vi "gugudan server.vi"() -> ()   [LabVIEW 2014]
uses:
  <vilib>/FTP/NI_FTP.lvlib
panel:
  in  "data 2":string="연결된 IP"
  in  "숫자형":dbl min=0.0 max=24.0 step=0.5
  in  "재시작":bool
  in  "2시간":bool
  in  "강제종료":bool
  in  "1시간":bool
  in  "종료취소":bool
  in  "종료":bool
  out "data":string="연결된 IP"
  in  "사용설명서":bool
  out "로그인":bool
  in  "ID":string="ID"
  in  "PW":string="PW"
  in  "E-Mail":string="E-Mail  address"
  out "참 거짓":string="상태창입니다."
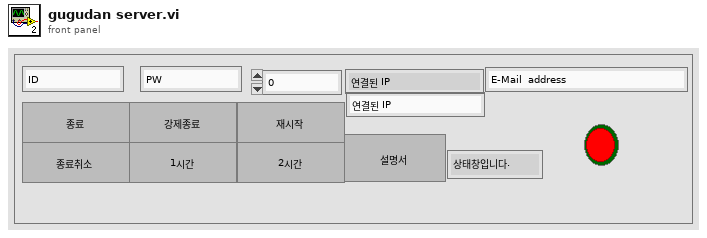
[diagram p1: front panel]
types:
  T1 = typedef "NI_FTP.lvlib/FTP Session.ctl" = refnum<k5>
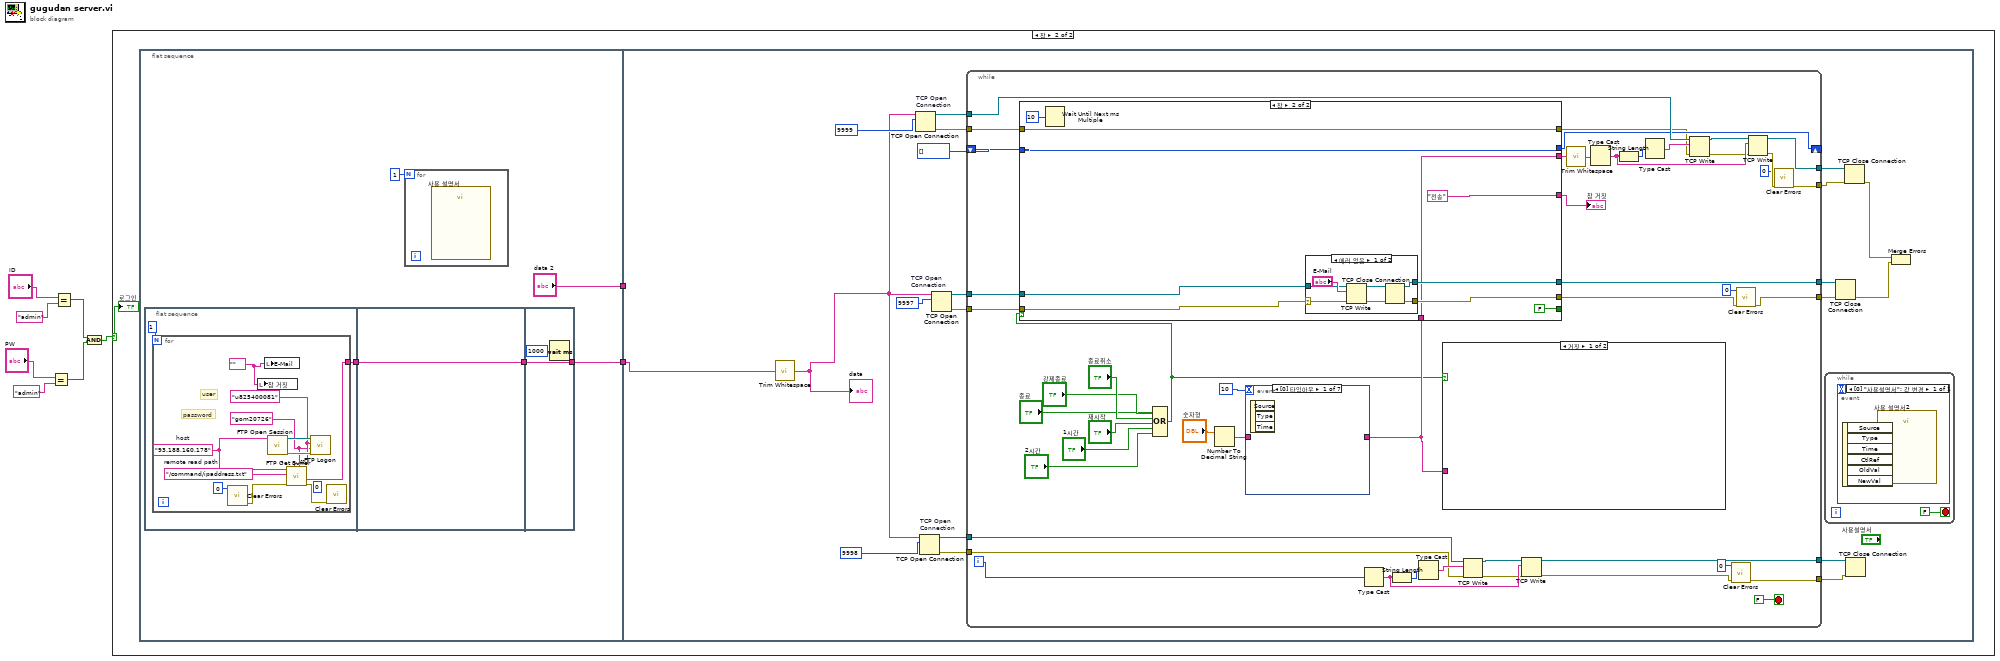
[diagram p0: block diagram]
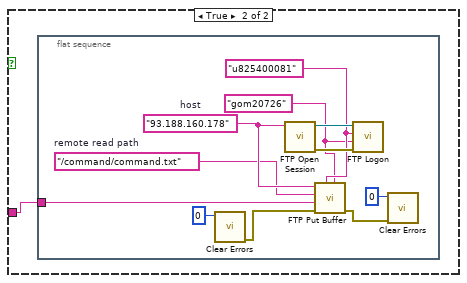
[diagram p3: hidden frame]
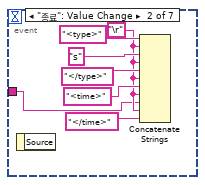
[diagram p4: hidden frame]
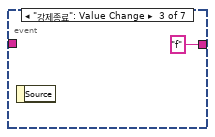
[diagram p5: hidden frame]
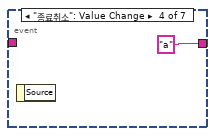
[diagram p6: hidden frame]
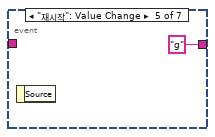
[diagram p7: hidden frame]
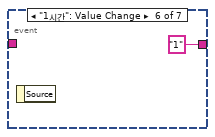
[diagram p8: hidden frame]
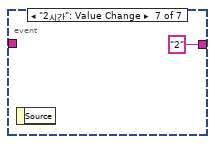
[diagram p9: hidden frame]
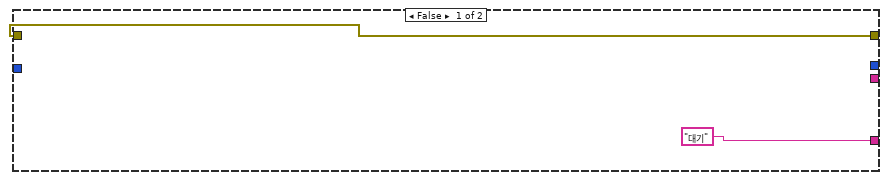
[diagram p10: hidden frame]
diagram:
  n1 = Equal?(x="PW", y="admin") -> (x = y?=w2:bool)
  n2 = Equal?(x="ID", y="admin") -> (x = y?=w3:bool)
  n3 = And(x=w3, y=w2) -> (x .and. y?=w1:bool)
  n4 = case shown="참" w1 {
    selector: w1 -> [_ w9]
    frame False {
    }
    frame True {
      n5 = flat-sequence {
        tunnel: [w14] -> w10
        tunnel: ["data 2"] -> w8
        tunnel: w10 -> [w32]
        tunnel: w8 -> [_]
        frame #0 {
          n6 = flat-sequence {
            tunnel: [w17] -> w13
            tunnel: w13 -> [w29]
            tunnel: [w29] -> w11
            tunnel: [w31] -> w14
            tunnel: w11 -> [w31]
            frame #0 {
              n7 = for {
                N: 1 -> [_]
                tunnel: [w18] -> w17
                (unwired) 0 ("specific error code to clear (0: all)")
                w24 = "gom20726"
                w25 = "u825400081"
                w22 = "/command/ipaddress.txt"  # remote read path
                w23 = "93.188.160.178"  # host
                w28 = ""
                # "user"
                # "password"
                n8 = call <vilib>:"Clear Errors.vi"("specific error code to clear (0: all)"=0) -> ("error out"=w21:errorcluster)  [unwired: 5 in, 1 out]
                n9 = local write "참 거짓"(w28) -> ()
                n10 = local write "E-Mail"(w28) -> ()
                n11 = call <vilib>:"FTP Open Session.vi"("address"=w23) -> ("error out"=w26:errorcluster, "ftp session"=w27:T1)  [unwired: 7 in, 2 out]
                n12 = call <vilib>:"FTP Get Buffer.vi"("password"=w24, "user"=w25, "error in (no error)"=w21, "remote path"=w22, "host"=w23) -> ("error out"=w19:errorcluster, "data"=w18:string)  [unwired: 4 in, 1 out]
                n13 = call <vilib>:"FTP Logon.vi"("error in (no error)"=w26, "password"=w24, "user"=w25, "ftp session"=w27) -> ()  [unwired: 4 in, 4 out]
                n14 = call <vilib>:"Clear Errors.vi"("error in (no error)"=w19) -> ()  [unwired: 5 in, 2 out]
              }
            }
            frame #1 {
            }
            frame #2 {
              n15 = Wait (ms)(milliseconds to wait=u32 1000 ("대기 시간(ms)")) -> ()  [unwired: 1 out]
            }
          }
          n16 = for {
            N: 1 -> [_]
            n17 = call "사용 설명서"() -> ()  [unwired: 10 in, 2 out]
          }
        }
        frame #1 {
          n18 = call <vilib>:"Trim Whitespace.vi"("string"=w32) -> ("trimmed string"=w33:string)  [unwired: 1 in]
          "data" <- w33
          n19 = TCP Open Connection "TCP Open \nConnection"(address=w33, remote port or service name=u16 9999) -> (connection ID=w51:refnum<k5>, error out=w47:errorcluster)  [unwired: 3 in]
          n20 = TCP Open Connection "TCP Open \nConnection"(address=w33, remote port or service name=u16 9998) -> (connection ID=w44:refnum<k5>, error out=w41:errorcluster)  [unwired: 3 in]
          n21 = TCP Open Connection "TCP Open \nConnection"(address=w33, remote port or service name=u16 9997 ("원격 포트 또는 서비스 이름")) -> (connection ID=w39:refnum<k5>, error out=w38:errorcluster)  [unwired: 3 in]
          n22 = while {
            tunnel: w51 -> [w97]
            tunnel: [w99] -> w49
            shift-right: [w92] -> _
            shift-left: i16[] [] -> [w98]
            tunnel: w47 -> [w91]
            tunnel: [w73] -> w35
            tunnel: w44 -> [w80]
            tunnel: [w79] -> w43
            tunnel: [w70] -> w42
            tunnel: w41 -> [w78]
            tunnel: [w67] -> w40
            tunnel: w39 -> [w76]
            tunnel: w38 -> [w75]
            tunnel: [w74] -> w36
            i -> [w77]
            stop <- FALSE stop-if-true
            n23 = Compound Arithmetic op=OR("종료", "강제종료", "종료취소", "재시작", "1시간", "2시간") -> (w53:bool)
            n24 = Number To Decimal String(number="숫자형") -> (decimal integer string=w56:string)  [unwired: 1 in]
            n25 = event shown="[0] 타임아웃" {
              selector: _ -> [_ _ _ _ _ _ _]
              dyn-events: _ -> [_ _ _ _ _ _ _]
              timeout: 10 -> [_ _ _ _ _ _ _]
              tunnel: w56 -> [_ w112 _ _ _ _ _]
              tunnel: [_ _ "f" "a" "g" "1" "2"] -> w54
              event Timeout {
                n26 = event-data() -> ()  [unwired: 1 in, 3 out]
              }
              event "종료": Value Change {
                w113 = "\r"
                n27 = event-data() -> ()  [unwired: 1 in, 1 out]
                n28 = Concatenate Strings("<type>", w113, "s", w113, "</type>", w113, "<time>", w113, w112, w113, "</time>") -> ()  [unwired: 1 out]
              }
              event "강제종료": Value Change {
                n29 = event-data() -> ()  [unwired: 1 in, 1 out]
              }
              event "종료취소": Value Change {
                n30 = event-data() -> ()  [unwired: 1 in, 1 out]
              }
              event "재시작": Value Change {
                n31 = event-data() -> ()  [unwired: 1 in, 1 out]
              }
              event "1시간": Value Change {
                n32 = event-data() -> ()  [unwired: 1 in, 1 out]
              }
              event "2시간": Value Change {
                n33 = event-data() -> ()  [unwired: 1 in, 1 out]
              }
            }
            n34 = case shown="참" w53 {
              tunnel: w98 -> [_ w135]
              tunnel: [_ w135] -> w92
              tunnel: [_ w126] -> w87
              tunnel: w91 -> [w125 w133]
              tunnel: [w125 w133] -> w90
              tunnel: ["대기" "전송"] -> w86
              tunnel: [_ FALSE ("불리언")] -> _
              tunnel: [_ w130] -> w66
              tunnel: w76 -> [_ w129]
              tunnel: w75 -> [_ w128]
              tunnel: [_ w127] -> w74
              tunnel: w54 -> [_ w126]
              frame False {
              }
              frame True {
                n35 = Wait Until Next ms Multiple(millisecond multiple=u32 10) -> ()  [unwired: 1 out]
                n36 = case shown="에러 없음" w128 {
                  selector: w128 -> [w138 w144]
                  tunnel: [w141 w143] -> w127
                  tunnel: [w140 w144] -> w130
                  tunnel: w129 -> [w136 w143]
                  frame No Error {
                    n37 = TCP Write(connection ID=w136, data in="E-Mail", error in (no error)=w138) -> (connection ID out=w142:refnum<k5>, error out=w139:errorcluster)  [unwired: 2 out]
                    n38 = TCP Close Connection(connection ID=w142, error in (no error)=w139) -> (connection ID out=w141:refnum<k5>, error out=w140:errorcluster)  [unwired: 1 out]
                  }
                  frame Error {
                  }
                }
              }
            }
            "참 거짓" <- w86
            n39 = Type Cast(x=w77) -> (*(type *) &x=w82:string)  [unwired: 1 in]
            n40 = String Length(string=w82) -> (length=w83:i32)
            n41 = Type Cast(x=w83) -> (*(type *) &x=w84:string)  [unwired: 1 in]
            n42 = case shown="거짓" w53 {
              tunnel: w54 -> [_ w100]
              frame False {
              }
              frame True {
                n43 = flat-sequence {
                  tunnel: w100 -> [w105]
                  frame #0 {
                    w108 = "gom20726"
                    w109 = "u825400081"
                    w106 = "/command/command.txt"  # remote read path
                    w107 = "93.188.160.178"  # host
                    n44 = call <vilib>:"Clear Errors.vi"("specific error code to clear (0: all)"=0) -> ("error out"=w103:errorcluster)  [unwired: 5 in, 1 out]
                    n45 = call <vilib>:"FTP Open Session.vi"("address"=w107) -> ("error out"=w110:errorcluster, "ftp session"=w111:T1)  [unwired: 7 in, 2 out]
                    n46 = call <vilib>:"FTP Put Buffer.vi"("password"=w108, "user"=w109, "error in (no error)"=w103, "data"=w105, "remote path"=w106, "host"=w107) -> ("error out"=w101:errorcluster)  [unwired: 4 in, 1 out]
                    n47 = call <vilib>:"FTP Logon.vi"("error in (no error)"=w110, "password"=w108, "user"=w109, "ftp session"=w111) -> ()  [unwired: 4 in, 4 out]
                    n48 = call <vilib>:"Clear Errors.vi"("error in (no error)"=w101, "specific error code to clear (0: all)"=0) -> ()  [unwired: 4 in, 2 out]
                  }
                }
              }
            }
            n49 = TCP Write(connection ID=w80, data in=w84, error in (no error)=w78) -> (connection ID out=w85:refnum<k5>, error out=w81:errorcluster)  [unwired: 1 in, 1 out]
            n50 = TCP Write(connection ID=w85, data in=w82, error in (no error)=w81) -> (connection ID out=w79:refnum<k5>, error out=w69:errorcluster)  [unwired: 1 in, 1 out]
            n51 = call <vilib>:"Trim Whitespace.vi"("string"=w87) -> ("trimmed string"=w88:string)  [unwired: 1 in]
            n52 = Type Cast(x=w88) -> (*(type *) &x=w93:string)  [unwired: 1 in]
            n53 = String Length(string=w93) -> (length=w94:i32)
            n54 = Type Cast(x=w94) -> (*(type *) &x=w95:string)  [unwired: 1 in]
            n55 = TCP Write(connection ID=w97, data in=w95, error in (no error)=w90) -> (connection ID out=w96:refnum<k5>, error out=w89:errorcluster)  [unwired: 1 in, 1 out]
            n56 = call <vilib>:"Clear Errors.vi"("error in (no error)"=w69, "specific error code to clear (0: all)"=0) -> ("error out"=w70:errorcluster)  [unwired: 4 in, 1 out]
            n57 = call <vilib>:"Clear Errors.vi"("error in (no error)"=w66, "specific error code to clear (0: all)"=0) -> ("error out"=w67:errorcluster)  [unwired: 4 in, 1 out]
            n58 = TCP Write(connection ID=w96, data in=w93, error in (no error)=w89) -> (connection ID out=w99:refnum<k5>, error out=w72:errorcluster)  [unwired: 1 in, 1 out]
            n59 = call <vilib>:"Clear Errors.vi"("error in (no error)"=w72, "specific error code to clear (0: all)"=0) -> ("error out"=w73:errorcluster)  [unwired: 4 in, 1 out]
          }
          n60 = while {
            stop <- FALSE stop-if-true
            n61 = event shown="[0] \"사용설명서\": 값 변경" {
              selector: _ -> [_]
              dyn-events: _ -> [_]
              timeout: _ -> [_]
              event "사용설명서": Value Change {
                n62 = event-data() -> ()  [unwired: 1 in, 6 out]
                n63 = call "사용 설명서2"() -> ()  [unwired: 10 in, 2 out]
              }
            }
          }
          n64 = TCP Close Connection(connection ID=w36, error in (no error)=w40) -> (error out=w34:errorcluster)  [unwired: 2 out]
          n65 = TCP Close Connection(connection ID=w49, error in (no error)=w35) -> (error out=w46:errorcluster)  [unwired: 1 in, 1 out]
          n66 = TCP Close Connection(connection ID=w43, error in (no error)=w42) -> ()  [unwired: 1 in, 2 out]
          n67 = Merge Errors(w46, w34) -> ()  [unwired: 1 out]
        }
      }
      "로그인" <- w9
    }
  }
